vi "Flow rate calc_Current1.vi"(9 "T venturi":fxp<+/-,42,16> format="%.31g", 10 "P venturi":fxp<+/-,42,16> format="%.31g") -> (1 "Flow rate g/s":dbl, 2 "Flow rate l/min":dbl)   [LabVIEW 2014]
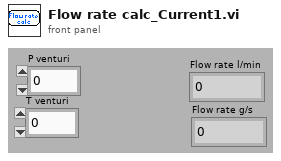
[diagram p1: front panel]
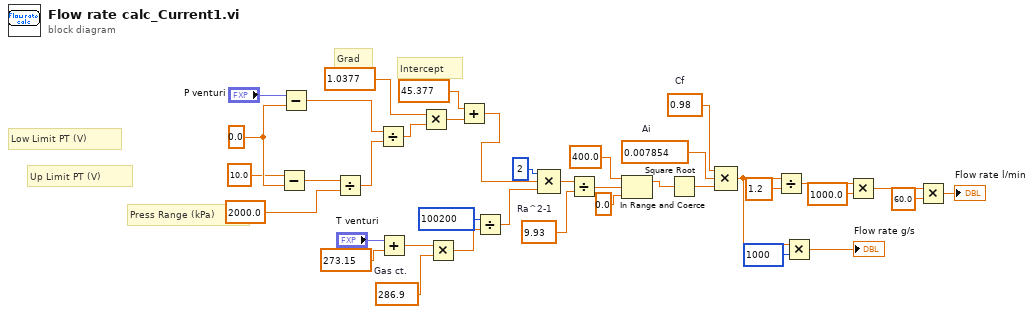
[diagram p0: block diagram]
diagram:
  w11 = 0.0 ("y")
  w32 = 9.93  # Ra^2-1
  w29 = 0.98  # Cf
  w35 = 286.9  # Gas ct.
  w30 = 0.007854  # Ai
  # "Intercept"
  # "Grad"
  # "Press Range (kPa)"
  # "Up Limit PT (V)"
  # "Low Limit PT (V)"
  n1 = Subtract(x=10.0, y=w11) -> (x-y=w9:dbl)
  n2 = Subtract(x="P venturi", y=w11) -> (x-y=w7:dbl)
  n3 = Divide(x=w9, y=2000.0) -> (x/y=w6:dbl)
  n4 = Divide(x=w7, y=w6) -> (x/y=w5:dbl)
  n5 = Add(x="T venturi", y=273.15) -> (x+y=w36:dbl)
  n6 = Multiply(x=1.0377, y=w5) -> (x*y=w4:dbl)
  n7 = Multiply(x=w36, y=w35) -> (x*y=w27:dbl)
  n8 = Add(x=45.377, y=w4) -> (x+y=w3:dbl)
  n9 = Divide(x=100200, y=w27) -> (x/y=w26:dbl)
  n10 = Compound Arithmetic op=MULTIPLY(2, w3, w26) -> (w33:dbl)
  n11 = Divide(x=w33, y=w32) -> (x/y=w16:dbl)
  n12 = In Range and Coerce(upper limit=400.0, x=w16, lower limit=0.0) -> (coerced(x)=w13:dbl)  [unwired: 1 out]
  n13 = Square Root(x=w13) -> (sqrt(x)=w31:dbl)
  n14 = Compound Arithmetic op=MULTIPLY(w29, w30, w31) -> (w23:dbl)
  n15 = Divide(x=w23, y=1.2) -> (x/y=w21:dbl)
  n16 = Multiply(x=w23, y=1000) -> (x*y=→"Flow rate g/s":dbl)
  n17 = Multiply(x=w21, y=1000.0) -> (x*y=w19:dbl)
  n18 = Multiply(x=w19, y=60.0) -> (x*y=→"Flow rate l/min":dbl)
